vi "Power Management.vi"(7 "I2C Channel":u8, 8 "error in (no error)":errorcluster, 9 "Operation Mode":enum16{"Read", "Write"}(ring), 10 "Power Management":T1 {"<PWR_MNG> Clock Select" items=["Internal Oscillator", "PLL with Gyro X Reference", "PLL with Gyro Y Reference", "PLL with Gyro Z Reference", "PLL with EXT 32.768KHz Reference", "PLL with EXT 19.2MHz Reference"]; "<PWR_MNG> Gyro Z Stanby Mode" items=["Gyro Z Standby ON"=8, "Gyro Z Standby OFF"=0]; "<PWR_MNG> Gyro Y Stanby Mode" items=["Gyro Y Standby ON"=16, "Gyro Y Standby OFF"=0]; "<PWR_MNG> Gyro X Stanby Mode" items=["Gyro X Standby ON"=32, "Gyro X Standby OFF"=0]; "<PWR_MNG> Low-Power Sleep Mode" items=["Put ITG3200 to Sleep"=64, "Wake Up ITG3200"=0]; "<PWR_MNG> HW Reset" items=["Hardware Reset OFF"=0, "Hadware Reset ON"=128]}, 11 "LINX Resource In":T2) -> (0 "error out":errorcluster, 2 "Power Management Register":T1 {"<PWR_MNG> Clock Select" items=["Internal Oscillator", "PLL with Gyro X Reference", "PLL with Gyro Y Reference", "PLL with Gyro Z Reference", "PLL with EXT 32.768KHz Reference", "PLL with EXT 19.2MHz Reference"]; "<PWR_MNG> Gyro Z Stanby Mode" items=["Gyro Z Standby ON"=8, "Gyro Z Standby OFF"=0]; "<PWR_MNG> Gyro Y Stanby Mode" items=["Gyro Y Standby ON"=16, "Gyro Y Standby OFF"=0]; "<PWR_MNG> Gyro X Stanby Mode" items=["Gyro X Standby ON"=32, "Gyro X Standby OFF"=0]; "<PWR_MNG> Low-Power Sleep Mode" items=["Put ITG3200 to Sleep"=64, "Wake Up ITG3200"=0]; "<PWR_MNG> HW Reset" items=["Hardware Reset OFF"=0, "Hadware Reset ON"=128]}, 3 "LINX Resource Out":T2)   [LabVIEW 2014, in "LMH-LINX.lvlib" / "ITG3200.lvlib"]
uses:
  <vilib>/MakerHub/LINX/Public/Sensors/Gyroscopes/ITG3200/ITG3200.lvlib
  <vilib>/MakerHub/LINX/Private/Type Defs/LINX Ref.ctl
  <vilib>/MakerHub/LINX/Private/Type Defs/Platform.ctl
  <vilib>/MakerHub/LINX/Private/Type Defs/Interface.ctl
  <vilib>/MakerHub/LINX/Private/Device/Type Defs/LINX Device Config.ctl
  <vilib>/MakerHub/LINX/Private/Device/Type Defs/TCP Config.ctl
  <vilib>/MakerHub/LINX/Private/Device/Type Defs/Channels.ctl
  <vilib>/MakerHub/LINX/Public/Sensors/Gyroscopes/ITG3200/Controls/Power_Management.ctl
  <vilib>/MakerHub/LINX/Private/Local IO/LinxI2cWrite.vi
  <vilib>/MakerHub/LINX/Public/Utilities/Check Channel.vi
  <vilib>/MakerHub/LINX/Private/Utilties/Generate Error.vi
  <vilib>/MakerHub/LINX/LMH-LINX.lvlib
  <vilib>/MakerHub/LINX/Private/Device/Device.lvlib
panel:
  # "INPUTS"
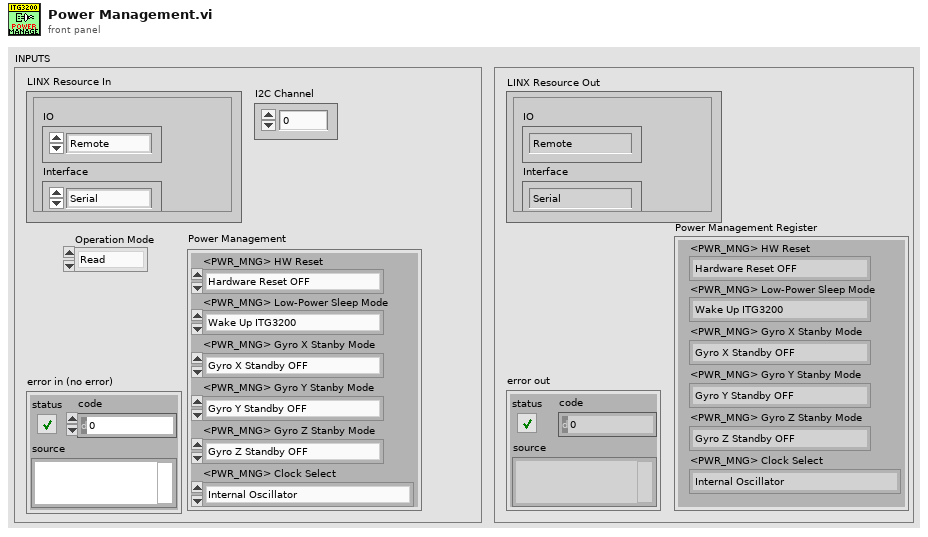
[diagram p1: front panel]
types:
  T1 = typedef "LMH-LINX.lvlib/ITG3200.lvlib/Power_Management.ctl" = cluster{"<PWR_MNG> HW Reset ":u8, "<PWR_MNG> Low-Power Sleep Mode":u8, "<PWR_MNG> Gyro X Stanby Mode":u8, "<PWR_MNG> Gyro Y Stanby Mode":u8, "<PWR_MNG> Gyro Z Stanby Mode":u8, "<PWR_MNG> Clock Select":u8}
  T2 = typedef "LMH-LINX.lvlib/LINX Ref.ctl" = cluster{"IO":T3, "Interface":T4, "LINX Device Config":T5}
  T3 = typedef "LMH-LINX.lvlib/Platform.ctl" = enum16{"Remote", "Local"}
  T4 = typedef "LMH-LINX.lvlib/Interface.ctl" = enum16{"Serial", "TCP"}
  T5 = typedef "LMH-LINX.lvlib/Device.lvlib/LINX Device Config.ctl" = cluster{"Interface":T4, "COM Port":refnum<visa-resource-name>, "TCP Configuration":T6, "Device Family":u8, "Device ID":u8, "Device Name":string, "TCP Ref":refnum<k5>, "Channels":T7}
  T6 = typedef "LMH-LINX.lvlib/Device.lvlib/TCP Config.ctl" = cluster{"IP Address":string, "Port":u16}
  T7 = typedef "LMH-LINX.lvlib/Channels.ctl" = cluster{"DI":u8[], "DO":u8[], "AI":u8[], "AO":u8[], "PWM":u8[], "QE":u8[], "UART":u8[], "I2C 2":u8[], "SPI":u8[], "CAN":u8[], "Servo":u8[], "AI Ref (V)":dbl, "AI Resolution (Bits)":u8, "AO Ref (V)":dbl, "AO Resolution (Bits)":u8}
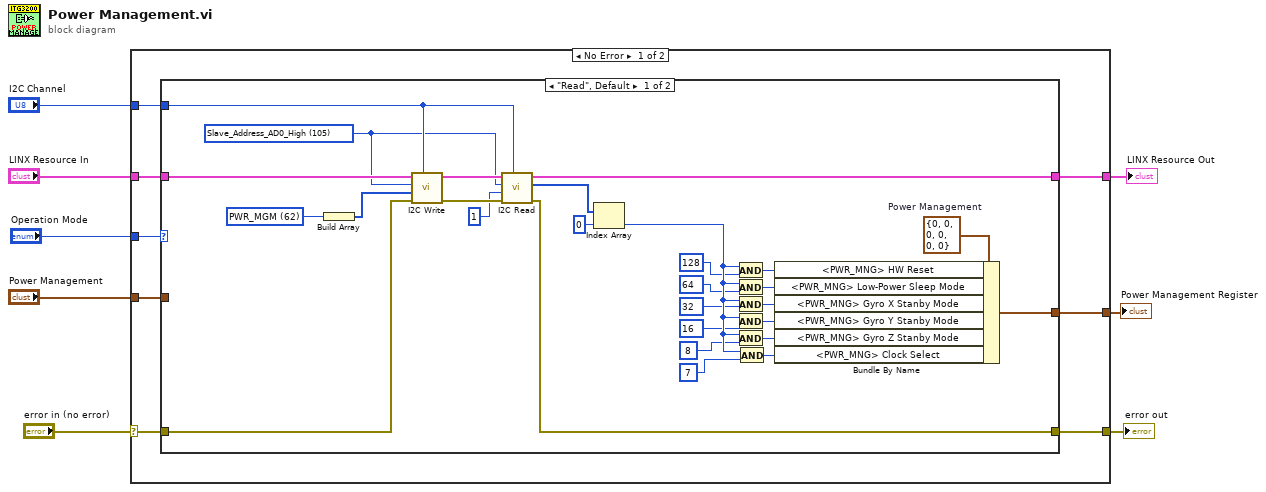
[diagram p0: block diagram]
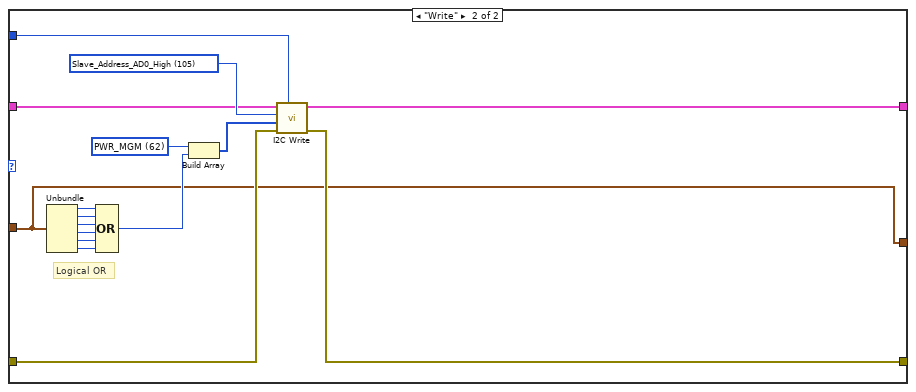
[diagram p2: hidden frame]
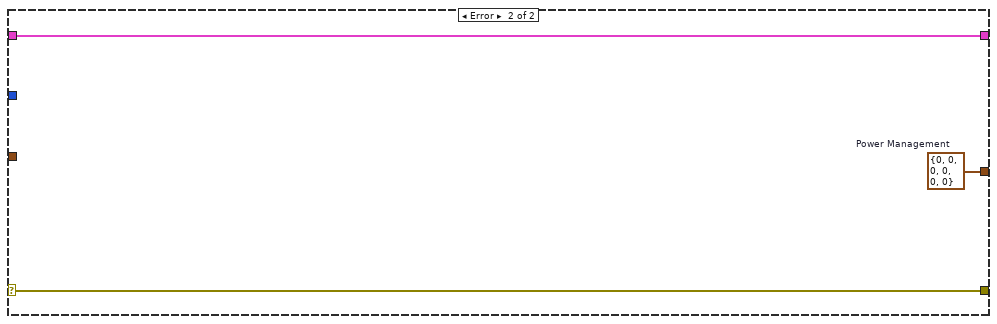
[diagram p3: hidden frame]
diagram:
  n1 = case shown="No Error" "error in (no error)" {
    selector: "error in (no error)" -> [w15 w63]
    tunnel: [w14 w63] -> w7
    tunnel: "LINX Resource In" -> [w16 w62]
    tunnel: "I2C Channel" -> [w12 _]
    tunnel: [w13 w62] -> w4
    tunnel: "Power Management" -> [w11 _]
    tunnel: "Operation Mode" -> [w10 _]
    tunnel: [w9 w61] -> w1
    frame No Error {
      n2 = case shown="\"Read\", Default" w10 {
        tunnel: w16 -> [w44 w56]
        tunnel: w15 -> [w43 w55]
        tunnel: [w42 w53] -> w14
        tunnel: [w41 w54] -> w13
        tunnel: w12 -> [w40 w57]
        tunnel: w11 -> [_ w45]
        tunnel: [w17 w45] -> w9
        frame "Read", Default {
          w31 = T1 {"<PWR_MNG> HW Reset "=0, "<PWR_MNG> Low-Power Sleep Mode"=0, "<PWR_MNG> Gyro X Stanby Mode"=0, "<PWR_MNG> Gyro Y Stanby Mode"=0, "<PWR_MNG> Gyro Z Stanby Mode"=0, "<PWR_MNG> Clock Select"=0}  # Power Management
          w39 = u8 62 items=["WHO_AM_I"=0, "SMPLRT_DIV"=21, "DLPF_FS"=22, "INT_CFG"=23, "INT_STATUS"=26, "TEMP_OUT_H"=27, "TEMP_OUT_L"=28, "GYRO_XOUT_H"=29, "GYRO_XOUT_L"=30, "GYRO_YOUT_H"=31, "GYRO_YOUT_L"=32, "GYRO_ZOUT_H"=33, "GYRO_ZOUT_L"=34, "PWR_MGM"=62] ("Register Map")
          w35 = u8 105 items=["Slave_Address_AD0_Low"=104, "Slave_Address_AD0_High"=105] ("Slave Addresses")
          n3 = Build Array(w39) -> (w38:u8[])
          n4 = call <vilib>:"I2C Write.vi"("I2C Channel"=w40, "Error In"=w43, "Data"=w38, "I2C Slave Address (0)"=w35, "LINX Resource"=w44) -> ("Error Out"=w36:errorcluster, "LINX Resource"=w37:T2)  [unwired: 5 in]
          n5 = call <vilib>:"I2C Read.vi"("I2C Channel"=w40, "Error In"=w36, "Bytes To Read"=u8 1, "I2C Slave Address (0)"=w35, "LINX Resource"=w37) -> ("Error Out"=w42:errorcluster, "Data"=w33:u8[], "LINX Resource"=w41:T2)  [unwired: 4 in]
          n6 = Index Array(array=w33, index=0) -> (element=w24:u8)
          n7 = And(x=w24, y=u8 128) -> (x .and. y?=w30:u8)
          n8 = And(x=w24, y=u8 64) -> (x .and. y?=w29:u8)
          n9 = And(x=w24, y=u8 32) -> (x .and. y?=w28:u8)
          n10 = And(x=w24, y=u8 16) -> (x .and. y?=w27:u8)
          n11 = And(x=w24, y=u8 8) -> (x .and. y?=w26:u8)
          n12 = And(x=w24, y=u8 7) -> (x .and. y?=w25:u8)
          n13 = Bundle By Name(cluster=w31, "<PWR_MNG> HW Reset"=w30, "<PWR_MNG> Low-Power Sleep Mode"=w29, "<PWR_MNG> Gyro X Stanby Mode"=w28, "<PWR_MNG> Gyro Y Stanby Mode"=w27, "<PWR_MNG> Gyro Z Stanby Mode"=w26, "<PWR_MNG> Clock Select"=w25) -> (w17:T1)
        }
        frame "Write" {
          w60 = u8 62 items=["WHO_AM_I"=0, "SMPLRT_DIV"=21, "DLPF_FS"=22, "INT_CFG"=23, "INT_STATUS"=26, "TEMP_OUT_H"=27, "TEMP_OUT_L"=28, "GYRO_XOUT_H"=29, "GYRO_XOUT_L"=30, "GYRO_YOUT_H"=31, "GYRO_YOUT_L"=32, "GYRO_ZOUT_H"=33, "GYRO_ZOUT_L"=34, "PWR_MGM"=62] ("Register Map")
          w58 = u8 105 items=["Slave_Address_AD0_Low"=104, "Slave_Address_AD0_High"=105] ("Slave Addresses")
          # "Logical OR"
          n14 = Unbundle(w45) -> ("<PWR_MNG> HW Reset"=w47:u8, "<PWR_MNG> Low-Power Sleep Mode"=w48:u8, "<PWR_MNG> Gyro X Stanby Mode"=w49:u8, "<PWR_MNG> Gyro Y Stanby Mode"=w50:u8, "<PWR_MNG> Gyro Z Stanby Mode"=w51:u8, "<PWR_MNG> Clock Select"=w52:u8)
          n15 = Compound Arithmetic op=OR(w47, w48, w49, w50, w51, w52) -> (w46:u8)
          n16 = Build Array(w60, w46) -> (w59:u8[])
          n17 = call <vilib>:"I2C Write.vi"("I2C Channel"=w57, "Error In"=w55, "Data"=w59, "I2C Slave Address (0)"=w58, "LINX Resource"=w56) -> ("Error Out"=w53:errorcluster, "LINX Resource"=w54:T2)  [unwired: 5 in]
        }
      }
    }
    frame Error {
      w61 = T1 {"<PWR_MNG> HW Reset "=0, "<PWR_MNG> Low-Power Sleep Mode"=0, "<PWR_MNG> Gyro X Stanby Mode"=0, "<PWR_MNG> Gyro Y Stanby Mode"=0, "<PWR_MNG> Gyro Z Stanby Mode"=0, "<PWR_MNG> Clock Select"=0}  # Power Management
    }
  }
  "error out" <- w7
  "LINX Resource Out" <- w4
  "Power Management Register" <- w1
